vi "TwoTanksModel_RealTime_regulator.vi"() -> ()   [LabVIEW 2020]
uses:
  <vilib>/Platform/TimedLoop/XDataNode/timing_clust.ctl
  <vilib>/Platform/TimedLoop/XDataNode/nitl_modes.ctl
  <vilib>/Platform/TimedLoop/XDataNode/wakeup.ctl
  <vilib>/Platform/TimedLoop/XDataNode/XDataNode.xnode
  <vilib>/Platform/TimedLoop/XDataNode/XDNodeRunTimeDep.lvlib
panel:
  out "H2 [cm]":dbl
  out "H1 [cm]":dbl
  in  "stop":bool
  out "Waveform Chart":cluster{"H [cm]":dbl, "H [cm]":dbl}(graph)
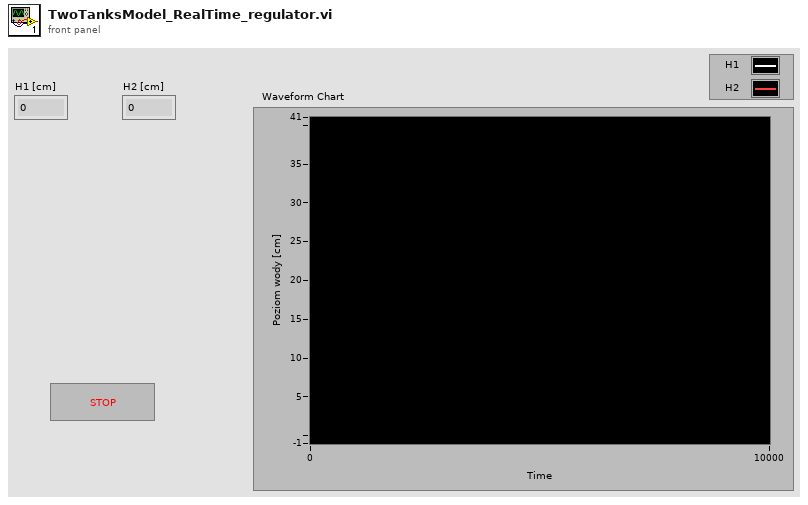
[diagram p1: front panel]
types:
  T1 = typedef "XDNodeRunTimeDep.lvlib/timing_clust.ctl" = cluster{"Expected End [f-1]":u64, "Actual End [f-1]":u64, "Finished Late? [f-1]":bool, "Expected End [i-1]":u64, "Actual End [i-1]":u64, "Finished Late? [i-1]":bool, "Expected Start [i]":u64, "Actual Start [i]":u64, "Expected Start [f]":u64, "Actual Start [f]":u64, "Source Name":string, "Structure Name":string, "Period":i64, "Deadline":i64, "Offset":i64, "Start":i64, "Priority":i32, "Timeout":i32, "Mode":T2, "Wakeup Reason":T3, "Error":errorcluster, "Source Type":string, "Secondary Source Type":string, "Global End Time":u64, "Global Start Time":u64, "Frame Duration":u64, "Iteration Duration":u64, "Assigned CPU":i32, "I/O Scan Engine Mode":u32}
  T2 = typedef "XDNodeRunTimeDep.lvlib/nitl_modes.ctl" = enum32{"No Change", "Process missed periods, maintain original phase", "Discard missed periods, maintain original phase", "Process missed periods, ignore original phase", "Discard missed periods, ignore original phase"}
  T3 = typedef "XDNodeRunTimeDep.lvlib/wakeup.ctl" = enum32{"Normal", "Aborted", "Asynchronous wakeup", "Timing source error", "Timed loop error", "Timeout"}
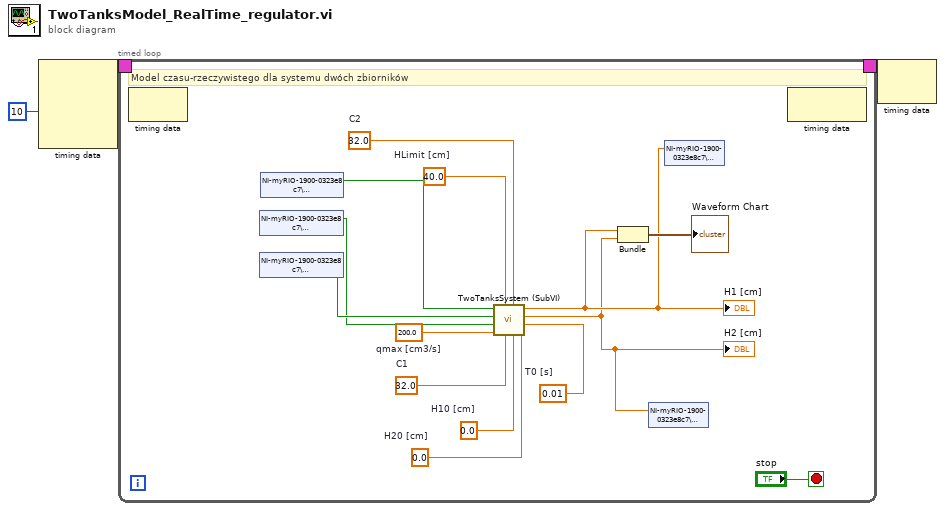
[diagram p0: block diagram]
diagram:
  n1 = node-c288(i64 10 ("Period")) -> (w3:T1)  [unwired: 3 in]
  n2 = timed-loop {
    timing: w3 -> [_]
    timing-out: [_] -> w2
    stop <- "stop" stop-if-true
    w15 = 0.01  # T0 [s]
    w9 = 32.0  # C2
    w12 = 32.0  # C1
    w14 = 0.0  # H20 [cm]
    w13 = 0.0  # H10 [cm]
    w10 = 40.0  # HLimit [cm]
    w11 = 200.0  # qmax [cm3/s]
    # "Model czasu-rzeczywistego dla systemu dwóch zbiorników"
    n3 = node-c288() -> ()  [unwired: 1 in, 1 out]
    n4 = shared-variable "NI-myRIO-1900-0323e8c7\\zmienneWspoldzielone.lvlib\\Zawor2"() -> (w5:bool)  [unwired: 1 in, 1 out]
    n5 = shared-variable "NI-myRIO-1900-0323e8c7\\zmienneWspoldzielone.lvlib\\Zawor1"() -> (w6:bool)  [unwired: 1 in, 1 out]
    n6 = shared-variable "NI-myRIO-1900-0323e8c7\\zmienneWspoldzielone.lvlib\\Pompa"() -> (w8:bool)  [unwired: 1 in, 1 out]
    n7 = call "TwoTanksSystem (SubVI).vi"("H20 [cm]"=w14, "T0 [s]"=w15, "H10 [cm]"=w13, "C2"=w9, "C1"=w12, "HLimit [cm]"=w10, "qmax [cm3/s]"=w11, "Valve2 On/Off"=w5, "Valve1 On/Off"=w6, "Pump On/Off"=w8) -> ("H2 [cm]"=w4:dbl, "H1 [cm]"=w7:dbl)
    "H1 [cm]" <- w7
    "H2 [cm]" <- w4
    n8 = Bundle("H1 [cm]"=w7, "H2 [cm]"=w4) -> (→"Waveform Chart":cluster{"H1 [cm]":dbl, "H2 [cm]":dbl})  [unwired: 1 in]
    n9 = shared-variable "NI-myRIO-1900-0323e8c7\\zmienneWspoldzielone.lvlib\\H2"(w4) -> ()  [unwired: 1 in, 1 out]
    n10 = shared-variable "NI-myRIO-1900-0323e8c7\\zmienneWspoldzielone.lvlib\\H1"(w7) -> ()  [unwired: 1 in, 1 out]
    n11 = node-c288() -> ()  [unwired: 1 in, 1 out]
  }
  n12 = node-c288(w2) -> ()  [unwired: 1 out]
